vi "2DStrArrayToEle.vi"(7 "Mothed":enum16{"init", "Get", "Set", "Close"}(ring), 8 "error in":errorcluster, 10 "AddrName":string, 11 "all rows":string[][](array[string])) -> (0 "error out":errorcluster, 1 "Address":u32, 2 "Array":u16[](array[numeric]), 3 "AddrData":string)   [LabVIEW 2016]
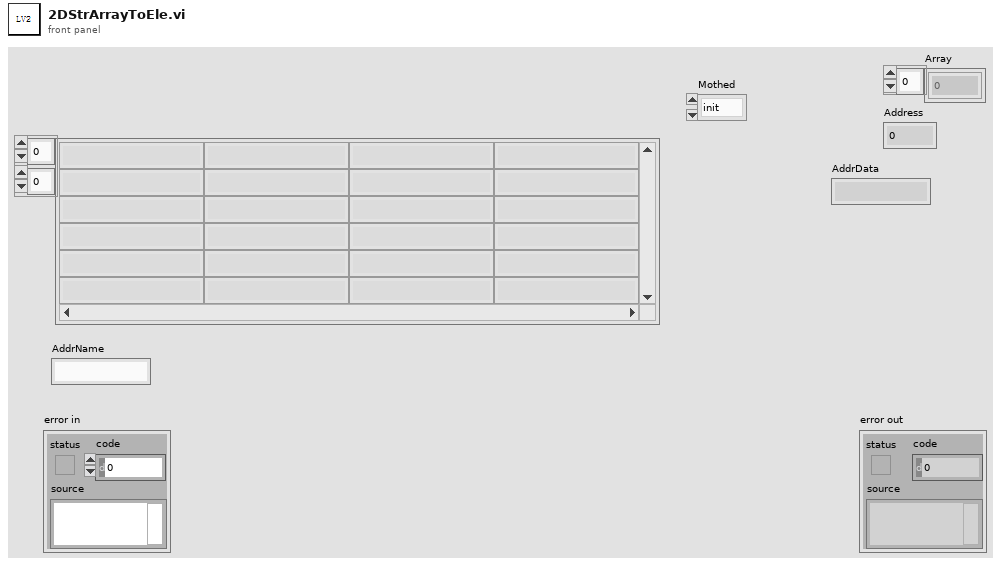
[diagram p1: front panel]
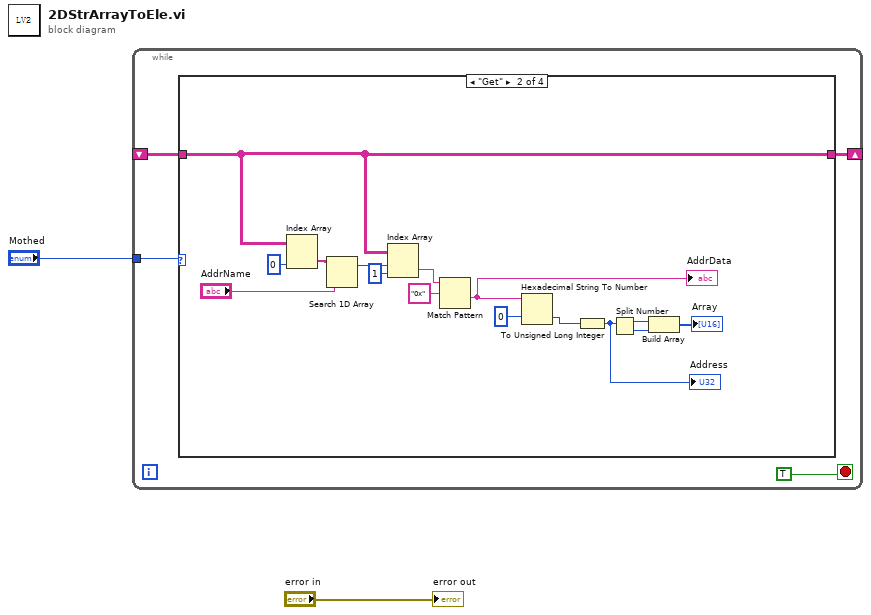
[diagram p0: block diagram]
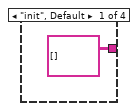
[diagram p2: hidden frame]
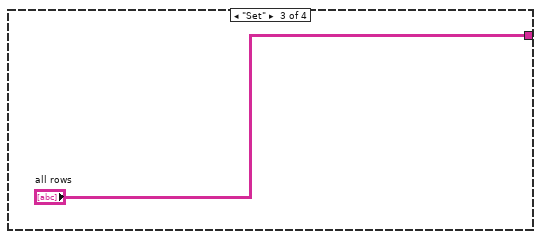
[diagram p3: hidden frame]
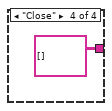
[diagram p4: hidden frame]
diagram:
  n1 = while {
    shift-right: [w4] -> _
    shift-left: _ -> [w3]
    tunnel: "Mothed" -> [w5]
    stop <- TRUE stop-if-true
    n2 = case shown="\"Get\"" w5 {
      tunnel: [string[][] [] ("all rows") w17 "all rows" string[][] [] ("all rows")] -> w4
      tunnel: w3 -> [_ w17 _ _]
      frame "init", Default {
      }
      frame "Get" {
        n3 = Index Array(array=w17, index (col)=0 ("index (row)")) -> (element=w20:string[])  [unwired: 1 in]
        n4 = Search 1D Array(1D array=w20, element="AddrName") -> (index of element=w18:i32)  [unwired: 1 in]
        n5 = Index Array(array=w17, index (row)=w18, index (col)=1 ("index (row)")) -> (element=w15:string)
        n6 = Match Pattern(string=w15, regular expression="0x") -> (after substring=w9:string)  [unwired: 1 in, 3 out]
        "AddrData" <- w9
        n7 = Hexadecimal String To Number(string=w9, default (0uL)=u32 0 ("default (0 I32)")) -> (number=w11:u32)  [unwired: 1 in, 1 out]
        n8 = To Unsigned Long Integer(number=w11) -> (unsigned 32bit integer=w14:u32)
        "Address" <- w14
        n9 = Split Number(x=w14) -> (hi(x)=w13:u16, lo(x)=w12:u16)
        n10 = Build Array(w13, w12) -> (→"Array":u16[])
      }
      frame "Set" {
      }
      frame "Close" {
      }
    }
  }
  "error out" <- "error in"
